vi "System Path.vi"(8 "error in (no error)":errorcluster caption="错误输入（无错误）", 11 "system directory type":T1 caption="系统目录类型" items=["用户目录"=0, "用户桌面"=1, "用户文档"=2, "用户应用程序数据"=3, "用户设置"=4, "用户临时目录"=5, "公共文档"=6, "公共应用程序数据"=7, "公共设置"=8, "公共缓存"=13, "系统核心库"=9, "系统安装库"=10, "应用程序文件"=11, "启动盘根目录"=12]) -> (0 "error out":errorcluster caption="错误输出", 3 "system directory":path caption="系统目录")   [LabVIEW 2012, in "Path Function.lvlib"]
uses:
  Path Function.lvlib
  <vilib>/Utility/sysdir.llb/System Directory Type.ctl
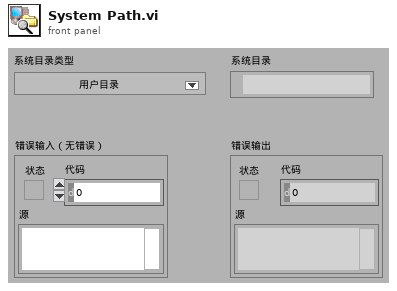
[diagram p1: front panel]
types:
  T1 = typedef "System Directory Type.ctl" = i32
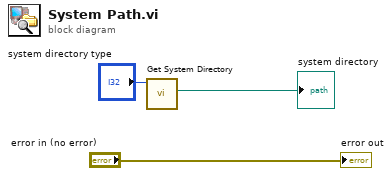
[diagram p0: block diagram]
diagram:
  n1 = call <vilib>:"Get System Directory.vi"("system directory type"="system directory type") -> ("system directory"=→"system directory":path)  [unwired: 10 in]
  "error out" <- "error in (no error)"
